vi "reset_table_tuned_by_user.vi"(8 "error in (no error)":errorcluster, 10 "NTable":u8, 11 "paramUnicorn in":T1) -> (0 "error out":errorcluster, 2 "cleaned_params":sgl[][](array[numeric]), 3 "paramUnicorn out":T1)   [LabVIEW 2017]
uses:
  Unicorn Labview Library/Control/unicorn_Param.ctl
  Unicorn Labview Library/Control/unicorn_conn.ctl
  Unicorn Labview Library/Control/unicorn_JSON.ctl
  Unicorn Labview Library/Control/unicorn_ParamInt.ctl
  Unicorn Labview Library/Control/unicorn_Telemetry.ctl
  Unicorn Labview Library/Control/unicorn_Table.ctl
  Unicorn Labview Library/Control/unicorn_ParamFloat.ctl
  Unicorn Labview Library/Unicorn Library.lvlib
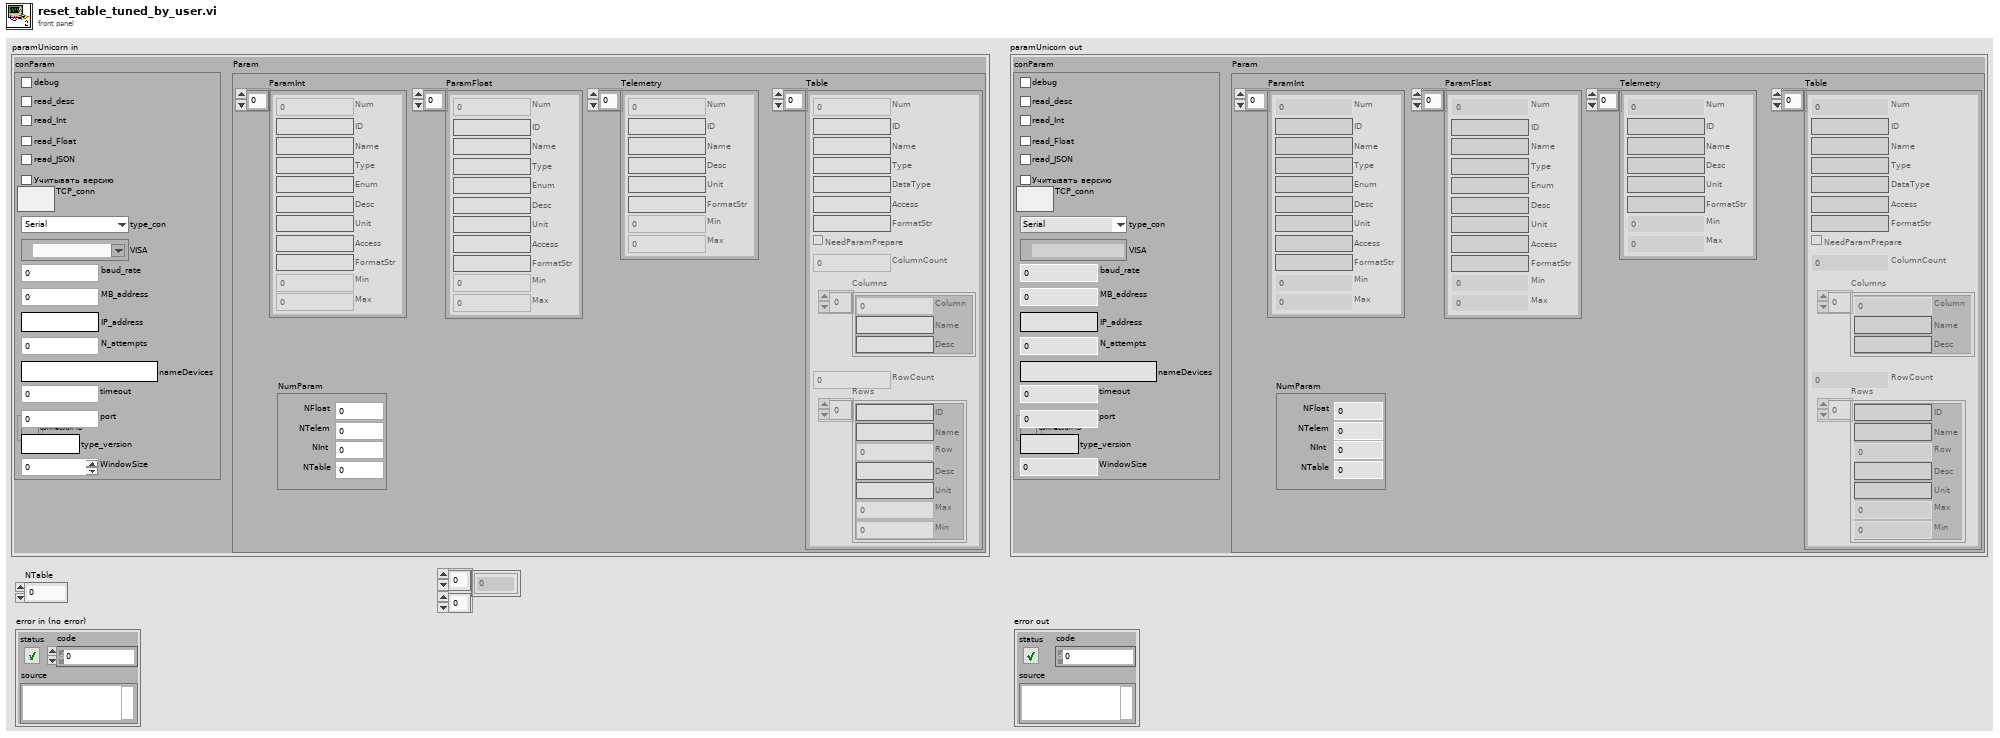
[diagram p1: front panel]
types:
  T1 = typedef "Unicorn Library.lvlib/unicorn_Param.ctl" = cluster{"conParam":T2, "Param":T3}
  T2 = typedef "Unicorn Library.lvlib/unicorn_conn.ctl" = cluster{"ReadIntParam":bool, "ReadDescrParam":bool, "ReadFloatParam":bool, "debug":bool, "ReadJSON":bool, "IP_address":string, "N_attempts":i32, "type_con":enum16{"Serial", "TCP"}, "MB_address":i32, "VISA":refnum<visa-resource-name>, "connection ID":refnum<k5>, "nameDevices":string, "timeout":i32, "port":u16, "type_version":string, "baud_rate":u32, "VersionControl":bool, "TCP_conn":bool, "WindowSize":i32}
  T3 = typedef "Unicorn Library.lvlib/unicorn_JSON.ctl" = cluster{"NumParam":cluster{"NTelem":i32, "NInt":i32, "NFloat":i32, "NTable":i32}, "ParamInt":T4, "Telemetry":T5, "Table":T6, "ParamFloat":T7}
  T4 = typedef "Unicorn Library.lvlib/unicorn_ParamInt.ctl" = cluster{"ID":string, "Num":i32, "Name":string, "Type":string, "Enum":string, "Desc":string, "Unit":string, "Access":string, "FormatStr":string, "Min":i32, "Max":i32}[]
  T5 = typedef "Unicorn Library.lvlib/unicorn_Telemetry.ctl" = cluster{"ID":string, "Num":i32, "Name":string, "Desc":string, "Unit":string, "FormatStr":string, "Min":i32, "Max":i32}[]
  T6 = typedef "Unicorn Library.lvlib/unicorn_Table.ctl" = cluster{"Num":i32, "Access":string, "ColumnCount":i32, "NeedParamPrepare":bool, "Columns":cluster{"Column":i32, "Desc":string, "Name":string}[], "DataType":string, "FormatStr":string, "ID":string, "Name":string, "RowCount":i32, "Rows":cluster{"Desc":string, "ID":string, "Max":i32, "Min":i32, "Name":string, "Row":i32, "Unit":string}[], "Type":string}[]
  T7 = typedef "Unicorn Library.lvlib/unicorn_ParamFloat.ctl" = cluster{"ID":string, "Num":i32, "Name":string, "Type":string, "Enum":string, "Desc":string, "Unit":string, "Access":string, "FormatStr":string, "Min":i32, "Max":i32}[]
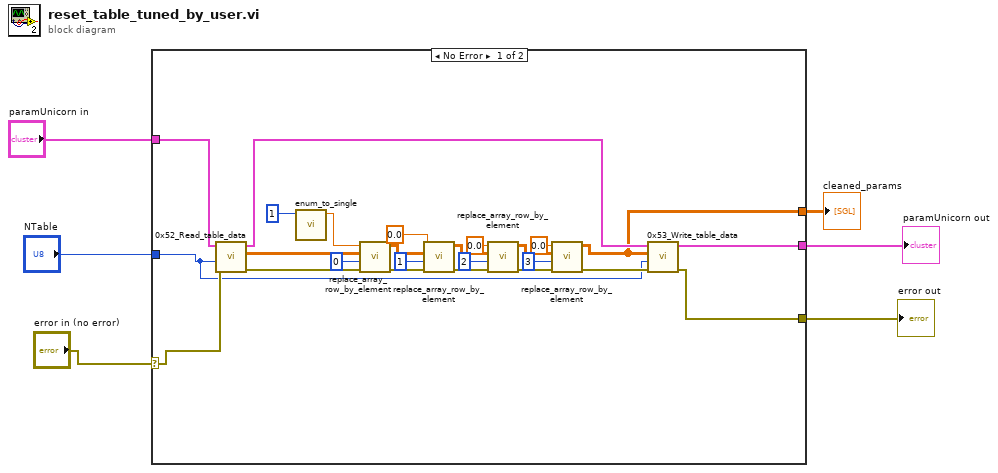
[diagram p0: block diagram]
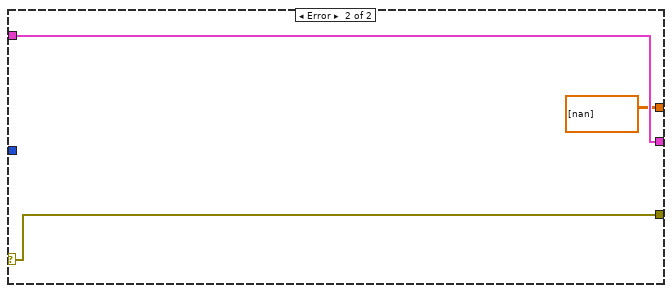
[diagram p2: hidden frame]
diagram:
  n1 = case shown="No Error" "error in (no error)" {
    selector: "error in (no error)" -> [w11 w34]
    tunnel: [w31 w34] -> w6
    tunnel: [w30 w33] -> w5
    tunnel: "NTable" -> [w10 _]
    tunnel: "paramUnicorn in" -> [w12 w33]
    tunnel: [w9 sgl[][] [[nan]] ("Array out")] -> w1
    frame No Error {
      n2 = call "0x52_Read_table_data.vi"("error in"=w11, "NTable"=w10, "paramUnicornIn"=w12) -> ("error out"=w14:errorcluster, "Array"=w13:sgl[][], "paramUnicornOut"=w28:T1)  [unwired: 6 in]
      n3 = call "enum_to_single.vi"("hi"=u8 1) -> ("Numeric"=w7:sgl)  [unwired: 10 in]
      n4 = call "replace_array_row_by_element.vi"("error_in"=w14, "index (row)"=0, "Array in"=w13, "element"=w7) -> ("error_out"=w25:errorcluster, "Array out"=w16:sgl[][])  [unwired: 6 in]
      n5 = call "replace_array_row_by_element.vi"("error_in"=w25, "index (row)"=1, "Array in"=w16, "element"=0.0) -> ("error_out"=w26:errorcluster, "Array out"=w17:sgl[][])  [unwired: 6 in]
      n6 = call "replace_array_row_by_element.vi"("error_in"=w26, "index (row)"=2, "Array in"=w17, "element"=0.0) -> ("error_out"=w27:errorcluster, "Array out"=w18:sgl[][])  [unwired: 6 in]
      n7 = call "replace_array_row_by_element.vi"("error_in"=w27, "index (row)"=3, "Array in"=w18, "element"=0.0) -> ("error_out"=w29:errorcluster, "Array out"=w9:sgl[][])  [unwired: 6 in]
      n8 = call "0x53_Write_table_data.vi"("error in"=w29, "Номер табличного параметра 2"=w10, "ArrayIn"=w9, "paramUnicorn"=w28) -> ("error out"=w31:errorcluster, "paramUnicorn 2"=w30:T1)  [unwired: 4 in, 2 out]
    }
    frame Error {
    }
  }
  "error out" <- w6
  "paramUnicorn out" <- w5
  "cleaned_params" <- w1
